vi "PC_NS_Signal get_signal_data.vi"(6 "Stop":refnum<vi>, 8 "error in (no error)":errorcluster, 11 "PC_NS_Signal in":refnum<class "PC_NS_Signal.lvclass">) -> (0 "error out":errorcluster, 3 "PC_NS_Signal out":refnum<class "PC_NS_Signal.lvclass">)   [LabVIEW 2018, in "PC_NS_Signal.lvclass"]
uses:
  PC_NS_Signal.lvclass
  PC_NS_Signal.lvclass/PC_NS_Signal.ctl
  <vilib>/Platform/TimedLoop/XDataNode/timing_clust.ctl
  <vilib>/Platform/TimedLoop/XDataNode/nitl_modes.ctl
  <vilib>/Platform/TimedLoop/XDataNode/wakeup.ctl
  <vilib>/Platform/TimedLoop/XDataNode/XDataNode.xnode
  <vilib>/Platform/TimedLoop/XDataNode/XDNodeRunTimeDep.lvlib
  <resource>/objmgr/ni.dex.rc
  <resource>/objmgr/ni.var.rc
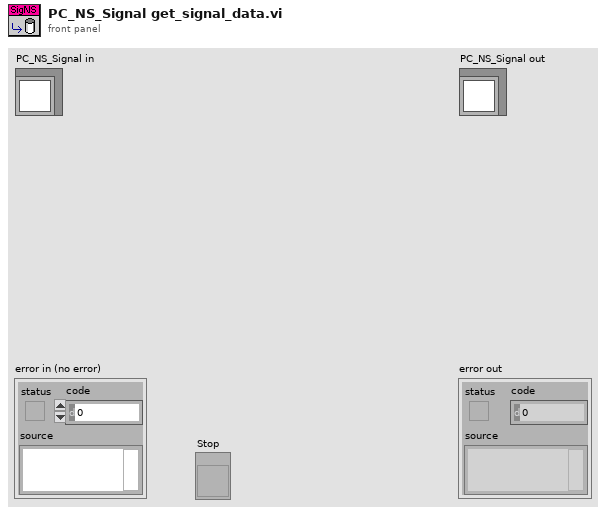
[diagram p1: front panel]
types:
  T1 = enum8{"Enabled", "Disabled", "Disabled and Grayed Out"}
  T2 = typedef "XDNodeRunTimeDep.lvlib/timing_clust.ctl" = cluster{"Expected End [f-1]":u64, "Actual End [f-1]":u64, "Finished Late? [f-1]":bool, "Expected End [i-1]":u64, "Actual End [i-1]":u64, "Finished Late? [i-1]":bool, "Expected Start [i]":u64, "Actual Start [i]":u64, "Expected Start [f]":u64, "Actual Start [f]":u64, "Source Name":string, "Structure Name":string, "Period":i64, "Deadline":i64, "Offset":i64, "Start":i64, "Priority":i32, "Timeout":i32, "Mode":T3, "Wakeup Reason":T4, "Error":errorcluster, "Source Type":string, "Secondary Source Type":string, "Global End Time":u64, "Global Start Time":u64, "Frame Duration":u64, "Iteration Duration":u64, "Assigned CPU":i32, "I/O Scan Engine Mode":u32}
  T3 = typedef "XDNodeRunTimeDep.lvlib/nitl_modes.ctl" = enum32{"No Change", "Process missed periods, maintain original phase", "Discard missed periods, maintain original phase", "Process missed periods, ignore original phase", "Discard missed periods, ignore original phase"}
  T4 = typedef "XDNodeRunTimeDep.lvlib/wakeup.ctl" = enum32{"Normal", "Aborted", "Asynchronous wakeup", "Timing source error", "Timed loop error", "Timeout"}
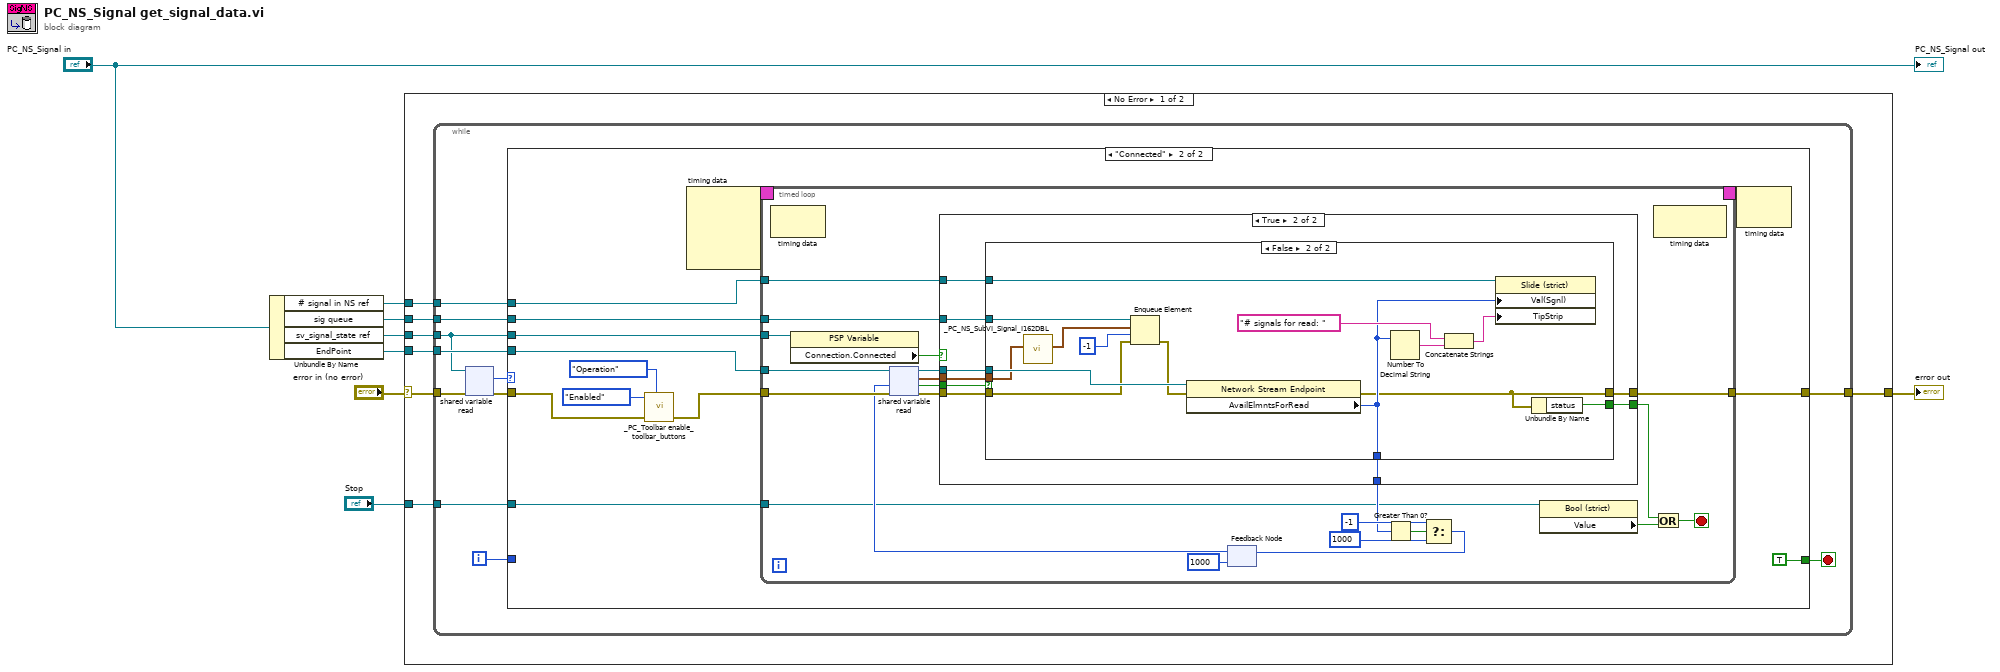
[diagram p0: block diagram]
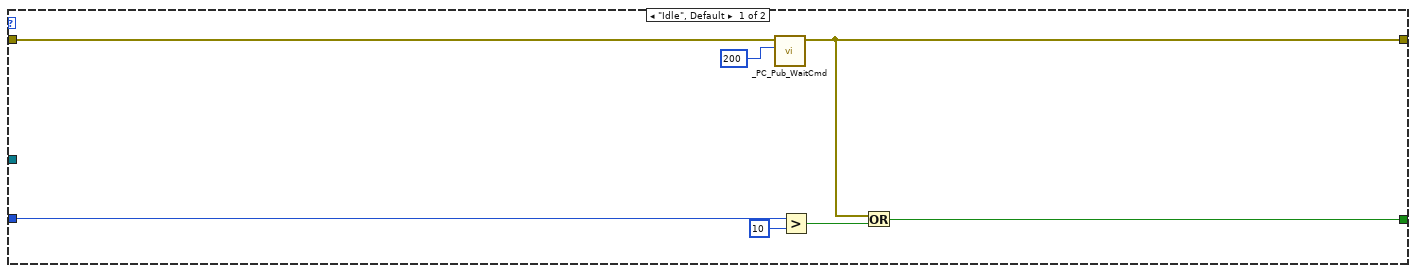
[diagram p2: hidden frame]
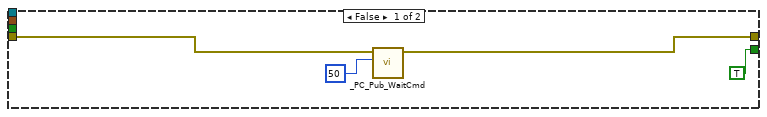
[diagram p3: hidden frame]
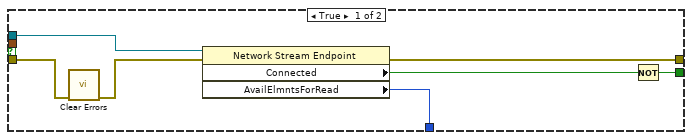
[diagram p4: hidden frame]
diagram:
  n1 = Unbundle By Name("PC_NS_Signal in") -> ("# signal in NS ref"=w5:refnum<vi>, "sig queue"=w4:refnum<queue>, "sv_signal_state ref"=w3:refnum<k21>, "EndPoint"=w8:refnum<k21>)
  n2 = case shown="No Error" "error in (no error)" {
    selector: "error in (no error)" -> [w10 w107]
    tunnel: w8 -> [w15 _]
    tunnel: [w14 w107] -> w7
    tunnel: w5 -> [w13 _]
    tunnel: w4 -> [w12 _]
    tunnel: w3 -> [w11 _]
    tunnel: "Stop" -> [w9 _]
    frame No Error {
      n3 = while {
        tunnel: w15 -> [w26]
        tunnel: w13 -> [w24]
        tunnel: w12 -> [w23]
        tunnel: w11 -> [w22]
        tunnel: w10 -> [w20]
        tunnel: [w25] -> w14
        tunnel: w9 -> [w16]
        i -> [w17]
        stop <- w18 stop-if-true
        n4 = shared-variable-read(w22, w20) -> (w19:errorcluster, w21:enum8{"Idle", "Init", "Connected", "Stop"})  [unwired: 1 out]
        n5 = case shown="\"Connected\"" w21 {
          tunnel: w26 -> [_ w44]
          tunnel: [w28 w43] -> w25
          tunnel: w24 -> [_ w42]
          tunnel: w23 -> [_ w41]
          tunnel: w22 -> [_ w40]
          tunnel: w19 -> [w31 w36]
          tunnel: [w27 TRUE] -> w18
          tunnel: w17 -> [w33 _]
          tunnel: w16 -> [_ w34]
          frame "Idle", Default {
            n6 = call "_PC_Pub_WaitCmd.vi"("milliseconds to wait"=u32 200, "error in (no error)"=w31) -> ("error out"=w28:errorcluster)  [unwired: 9 in]
            n7 = Greater?(x=w33, y=10) -> (0:w29:bool)
            n8 = Or(x=w28, y=w29) -> (x .or. y?=w27:bool)
          }
          frame "Connected" {
            n9 = call "_PC_Toolbar enable_toolbar_buttons.vi"("Disabled"=T1."Enabled", "Function"=enum16{"Save reference", "Operation"}."Operation", "error in (no error)"=w36) -> ("error out"=w35:errorcluster)  [unwired: 6 in]
            n10 = node-c288() -> (w46:T2)  [unwired: 4 in]
            n11 = timed-loop {
              tunnel: w44 -> [w60]
              tunnel: w35 -> [w68]
              tunnel: [w58] -> w43
              tunnel: w42 -> [w59]
              timing: w46 -> [_]
              timing-out: [_] -> w45
              tunnel: w41 -> [w61]
              tunnel: w40 -> [w52]
              tunnel: w34 -> [w50]
              stop <- w47 stop-if-true
              n12 = node-c288() -> ()  [unwired: 1 in, 1 out]
              n13 = property class="PSP Variable"(reference=w52) -> ("Connection.Connected"=w51:bool)  [unwired: 1 in, 2 out]
              n14 = feedback #1(1000 ("f")) -> (w63:i32)
              n15 = shared-variable-read(w60, w68, w63) -> (w67:refnum<k21>, w53:errorcluster, w54:bool, w55:waveform(i16))
              n16 = case shown="True" w51 {
                tunnel: w67 -> [_ w81]
                tunnel: w61 -> [_ w80]
                tunnel: w59 -> [_ w79]
                tunnel: [w70 w75] -> w58
                tunnel: [_ w78] -> w57
                tunnel: w55 -> [_ w77]
                tunnel: w53 -> [w69 w73]
                tunnel: w54 -> [_ w76]
                tunnel: [TRUE ("status") w74] -> w48
                frame False {
                  n17 = call "_PC_Pub_WaitCmd.vi"("milliseconds to wait"=u32 50, "error in (no error)"=w69) -> ("error out"=w70:errorcluster)  [unwired: 9 in]
                }
                frame True {
                  n18 = case shown="False" w76 {
                    tunnel: w81 -> [w88 w102]
                    tunnel: w80 -> [_ w101]
                    tunnel: w77 -> [_ w94]
                    tunnel: w79 -> [_ w95]
                    tunnel: [w86 w91] -> w75
                    tunnel: [w87 w96] -> w78
                    tunnel: [w82 w90] -> w74
                    tunnel: w73 -> [w84 w89]
                    frame True {
                      n19 = call <vilib>:"Clear Errors.vi"("error in (no error)"=w84) -> ("error out"=w83:errorcluster)  [unwired: 5 in, 1 out]
                      n20 = property class="Network Stream Endpoint"(reference=w88, error in=w83) -> (error out=w86:errorcluster, "Connected"=w85:bool, "AvailElmntsForRead"=w87:i32)  [unwired: 1 out]
                      n21 = Not(x=w85) -> (.not. x?=w82:bool)
                    }
                    frame False {
                      n22 = call "_PC_NS_SubVI_Signal_I162DBL.vi"("Int signal in"=w94) -> ("SGL sigal out"=w93:waveform(sgl))  [unwired: 9 in, 1 out]
                      n23 = Enqueue Element(queue=w101, element=w93, timeout in ms (-1)=-1, error in (no error)=w89) -> (error out=w100:errorcluster)  [unwired: 2 out]
                      n24 = property class="Network Stream Endpoint"(reference=w102, error in=w100) -> (error out=w91:errorcluster, "AvailElmntsForRead"=w96:i32)  [unwired: 1 out]
                      n25 = Number To Decimal String(number=w96) -> (decimal integer string=w97:string)  [unwired: 1 in]
                      n26 = Concatenate Strings("# signals for read: ", w97) -> (w99:string)
                      n27 = property class="Slide (strict)"(reference=w95, "Val(Sgnl)"=w96, "TipStrip"=w99) -> ()  [unwired: 1 in, 2 out]
                      n28 = Unbundle By Name(w91) -> ("status"=w90:bool)
                    }
                  }
                }
              }
              n29 = Greater Than 0?(x=w57) -> (x > 0?=w66:bool)
              n30 = Select(t=-1 ("timeout ms (-1)"), s=w66, f=1000) -> (s? t:f=w64:i32)
              n31 = feedback-in #1(w64) -> ()
              n32 = property class="Bool (strict)"(reference=w50) -> ("Value"=w49:bool)  [unwired: 1 in, 2 out]
              n33 = node-c288() -> ()  [unwired: 1 in, 1 out]
              n34 = Or(x=w48, y=w49) -> (x .or. y?=w47:bool)
            }
            n35 = node-c288(w45) -> ()  [unwired: 1 out]
          }
        }
      }
    }
    frame Error {
    }
  }
  "error out" <- w7
  "PC_NS_Signal out" <- "PC_NS_Signal in"
